vi "Test 4 Ex 2.vi"(8 "error in (no error)":errorcluster, 11 "Test Case In":refnum<class "Day X Test.lvclass">) -> (0 "error out":errorcluster, 3 "Test Case Out":refnum<class "Day X Test.lvclass">)   [LabVIEW 2020, in "Day X Test.lvclass"]
uses:
  Day X Test.lvclass
  C:/Program Files (x86)/National Instruments/LabVIEW 2020/vi.lib/Astemes/LUnit/Test Case.lvclass
  <vilib>/Astemes/LUnit/Test Case.lvclass/Test Case.ctl
  4993e8ee-a06a-463a-9684-69129f64d5ce.vi
  <vilib>/Astemes/LUnit/Append Pass Result.vi
  <vilib>/Astemes/LUnit/Append Fail Result.vi
  <vilib>/Astemes/LUnit/Describe Comparison.vi
  <vilib>/Astemes/LUnit/Compare Variants.vi
  <vilib>/Astemes/LUnit/Variant to string.vi
  <vilib>/Utility/Data Type/Get Type Information.vi
  <vilib>/Utility/LVClass/Get LV Class Name.vi
  Galaxy/Galaxy.lvclass
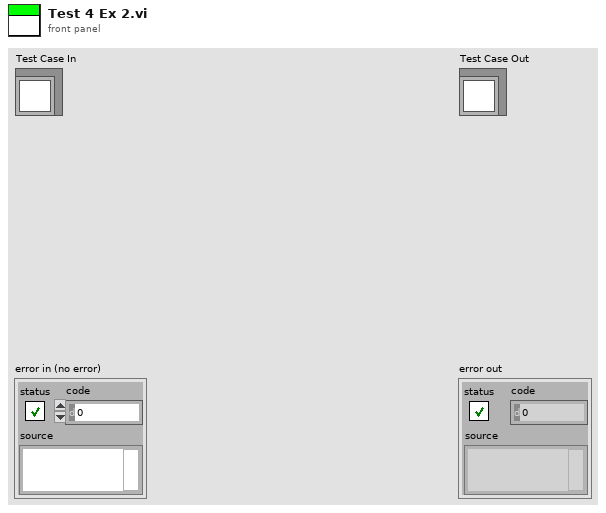
[diagram p1: front panel]
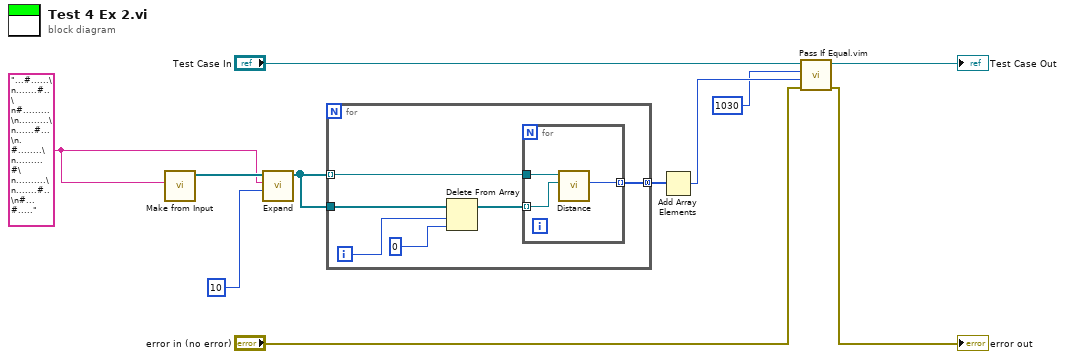
[diagram p0: block diagram]
diagram:
  w6 = "...#......\n.......#..\n#.........\n..........\n......#...\n.#........\n.........#\n..........\n.......#..\n#...#....." ("Input")
  n1 = call "Make from Input.vi"("Input"=w6) -> ("Galaxy out"=w7:refnum<class "Galaxy.lvclass">[])  [unwired: 9 in, 1 out]
  n2 = call "Expand.vi"("Factor"=10, "Input"=w6, "Galaxy in"=w7) -> ("Array"=w5:refnum<class "Galaxy.lvclass">[])  [unwired: 7 in, 1 out]
  n3 = for {
    tunnel: w5 -> [w17] mode=indexing
    tunnel: w5 -> [w16]
    tunnel: [w12] -> w4 mode=concatenating
    i -> [w15]
    n4 = Delete From Array(array=w16, length=w15, index=0) -> (array with subset deleted=w13:refnum<class "Galaxy.lvclass">[])  [unwired: 1 out]
    n5 = for {
      tunnel: w17 -> [w20]
      tunnel: w13 -> [w19] mode=indexing
      tunnel: [w18] -> w12 mode=indexing
      n6 = call "Distance.vi"("Galaxy in 2"=w19, "Galaxy in"=w20) -> ("Numeric"=w18:u64)  [unwired: 8 in, 1 out]
    }
  }
  n7 = Add Array Elements(numeric array=w4) -> (sum=w2:u64)
  n8 = call "Pass If Equal.vim"("error in (no error)"="error in (no error)", "Actual"=w2, "Expected"=u64 1030 ("sum"), "LUnit Test Case In"="Test Case In") -> ("error out"=→"error out":errorcluster, "LUnit Test Case Out"=→"Test Case Out":refnum<class "Day X Test.lvclass">)  [unwired: 6 in]
